vi "PH_Sixpack.read Database.vi"(0 "DB Entry to read":string, 1 "error in (no error)":errorcluster) -> (2 "COM Port":string, 3 "SixPack ID":string, 4 "Ignore Error":string, 5 "error out":errorcluster)   [LabVIEW 2014, in "PH_Sixpack.lvlib"]
uses:
  PH_Sixpack.lvlib
  PH_Basics/PH_Common/PH_Common.lvlib
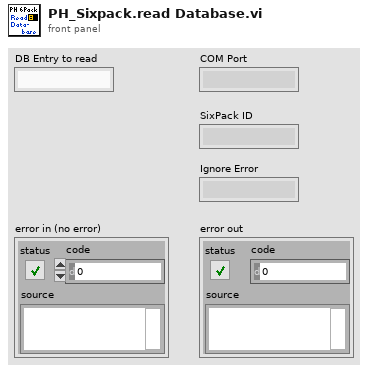
[diagram p1: front panel]
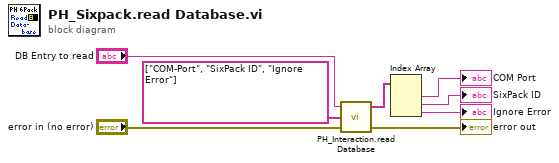
[diagram p0: block diagram]
diagram:
  n1 = call "PH_Interaction.read Database.vi"("error in (no error)"="error in (no error)", "Strings to search for"=string[] ["COM-Port", "SixPack ID", "Ignore Error"] ("Strings to search for in"), "DB Entry to read"="DB Entry to read") -> ("error out"=→"error out":errorcluster, "Values"=w7:string[])  [unwired: 1 in]
  n2 = Index Array(array=w7) -> (element #1=→"COM Port":string, element #2=→"SixPack ID":string, element #3=→"Ignore Error":string)  [unwired: 3 in]
